vi "writeToXML.vi"(8 "error in (no error)":errorcluster, 10 "Class Label":string="azElTracking", 11 "AzElTracking in":refnum<class "AzElTracking.lvclass">) -> (0 "error out":errorcluster, 2 "XML out":string="<AzElTracking>\n  <azimuthDemandedPosition>0</azimuthDemandedPosition>\n  <azVelocity>0</azVelocity>\n  <cableWrapDesired>C</cableWrapDesired>\n  <elevationDemandedPosition>0</elevationDemandedPosition>\n  <elVelocity>0</elVelocity>\n  <time>0</time>\n</AzElTracking>", 3 "AzElTracking out":refnum<class "AzElTracking.lvclass">)   [LabVIEW 2022 SP3, in "TCSDataDefinitions.lvlib" / "TCSMountControlStatus.lvlib" / "AzElTracking.lvclass"]
uses:
  AzElTracking.lvclass
  <userlib>/Common/UnitsAndXML/FlattenItemWithUnitToXML/FlattenPlaneAngleToXML/PlaneAngleUnit.ctl
  <userlib>/Common/UnitsAndXML/FlattenItemWithUnitToXML/FlattenAngularVelocityToXML/AngularVelocityUnit.ctl
  <userlib>/Common/UnitsAndXML/FlattenItemWithUnitToXML/FlattenTimeToXML/TimeUnit.ctl
  AzElTracking.lvclass/AzElTracking.ctl
  <userlib>/Common/UnitsAndXML/UnitsAndXML.lvlib
  <userlib>/Common/XML/XMLGenerator/XMLGenerator.lvclass
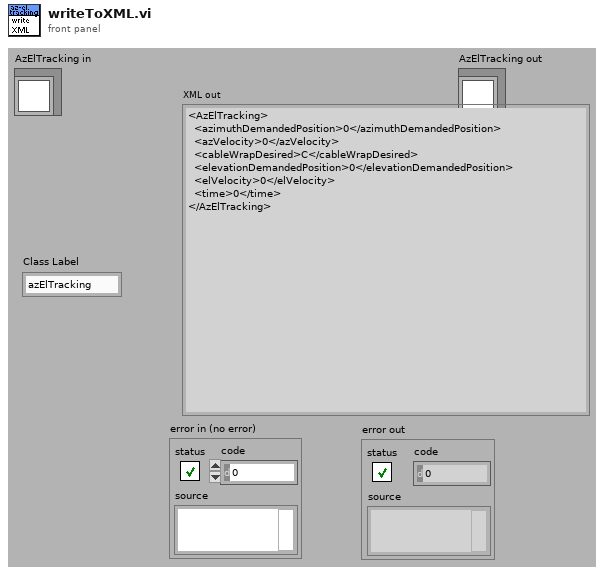
[diagram p1: front panel]
types:
  T1 = typedef "UnitsAndXML.lvlib/TimeUnit.ctl" = enum16{"s", "d", "h", "min", "a"}
  T2 = typedef "UnitsAndXML.lvlib/AngularVelocityUnit.ctl" = enum16{"\"/a", "deg/s", "\"/s"}
  T3 = typedef "UnitsAndXML.lvlib/PlaneAngleUnit.ctl" = enum16{"rad", "deg", "'", "\""}
  T4 = typedef "TCSDataDefinitions.lvlib/TCSMountControlStatus.lvlib/CableWrapDesired.ctl" = enum16{"C", "W", "S"}
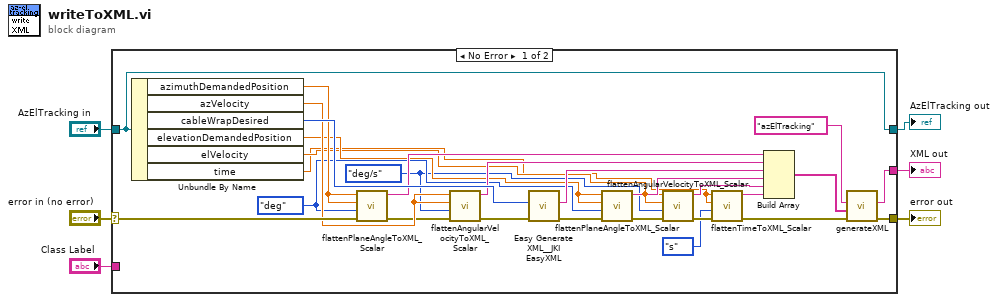
[diagram p0: block diagram]
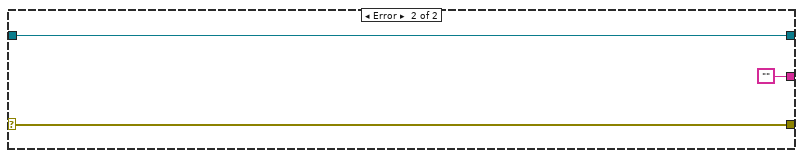
[diagram p2: hidden frame]
diagram:
  n1 = case shown="No Error" "error in (no error)" {
    selector: "error in (no error)" -> [w27 w36]
    tunnel: [w30 w36] -> w5
    tunnel: [w8 w35] -> w3
    tunnel: "AzElTracking in" -> [w8 w35]
    tunnel: [w29 ""] -> w2
    tunnel: "Class Label" -> [_ _]
    frame No Error {
      w16 = AngularVelocityUnit."deg/s" ("angularVelocityUnitInXML")
      w21 = PlaneAngleUnit."deg" ("planeAngleUnitInXML")
      n2 = Unbundle By Name(w8) -> ("azimuthDemandedPosition"=w28:dbl[unit], "azVelocity"=w25:dbl[unit], "cableWrapDesired"=w33:T4, "elevationDemandedPosition"=w20:dbl[unit], "elVelocity"=w17:dbl[unit], "time"=w10:dbl[unit])
      n3 = call <userlib>:"flattenPlaneAngleToXML_Scalar.vi"("error in (no error)"=w27, "planeAngleUnitInXML"=w21, "planeAngleAgain"=w28, "planeAngle"=w28) -> ("error out"=w24:errorcluster, "xmlString"=w26:string)  [unwired: 6 in]
      n4 = call <userlib>:"flattenAngularVelocityToXML_Scalar.vi"("error in (no error)"=w24, "angularVelocityUnitInXML"=w16, "anuglarVelocityAgain"=w25, "angularVelocity"=w25) -> ("error out"=w22:errorcluster, "xmlString"=w23:string)  [unwired: 6 in]
      n5 = call <vilib>:"Easy Generate XML__JKI EasyXML.vi"("error in (no error)"=w22, "LabVIEW Data"=w33) -> ("error out"=w19:errorcluster, "XML String"=w32:string)  [unwired: 8 in]
      n6 = call <userlib>:"flattenPlaneAngleToXML_Scalar.vi"("error in (no error)"=w19, "planeAngleUnitInXML"=w21, "planeAngleAgain"=w20, "planeAngle"=w20) -> ("error out"=w15:errorcluster, "xmlString"=w18:string)  [unwired: 6 in]
      n7 = call <userlib>:"flattenAngularVelocityToXML_Scalar.vi"("error in (no error)"=w15, "angularVelocityUnitInXML"=w16, "anuglarVelocityAgain"=w17, "angularVelocity"=w17) -> ("error out"=w14:errorcluster, "xmlString"=w11:string)  [unwired: 6 in]
      n8 = call <userlib>:"flattenTimeToXML_Scalar.vi"("error in (no error)"=w14, "timeUnitInXML"=TimeUnit."s", "timeAgain"=w10, "time"=w10) -> ("error out"=w13:errorcluster, "xmlString"=w12:string)  [unwired: 6 in]
      n9 = Build Array(w26, w23, w32, w18, w11, w12) -> (w31:string[])
      n10 = call <userlib>:"generateXML.vi"("error in"=w13, "childrenXML"=w31, "elementName"="azElTracking" ("Class Label")) -> ("error out"=w30:errorcluster, "XML out"=w29:string)  [unwired: 6 in, 1 out]
    }
    frame Error {
    }
  }
  "error out" <- w5
  "AzElTracking out" <- w3
  "XML out" <- w2
